vi "ConfigXMLCore.vi"(9 "ConnectionData":T1, 10 "controlsToSave":refnum<vi>[](array[refnum]), 11 "ConfigXMLControl":T2) -> ()   [LabVIEW 2015]
uses:
  ConfigXMLControl.ctl
  General/RemoteFiles/connectionData.ctl
panel:
  out "robotIP":string
  # "Core controller VI for the XML config plugin.\nhandles all saving, loading, file transfer, etc."
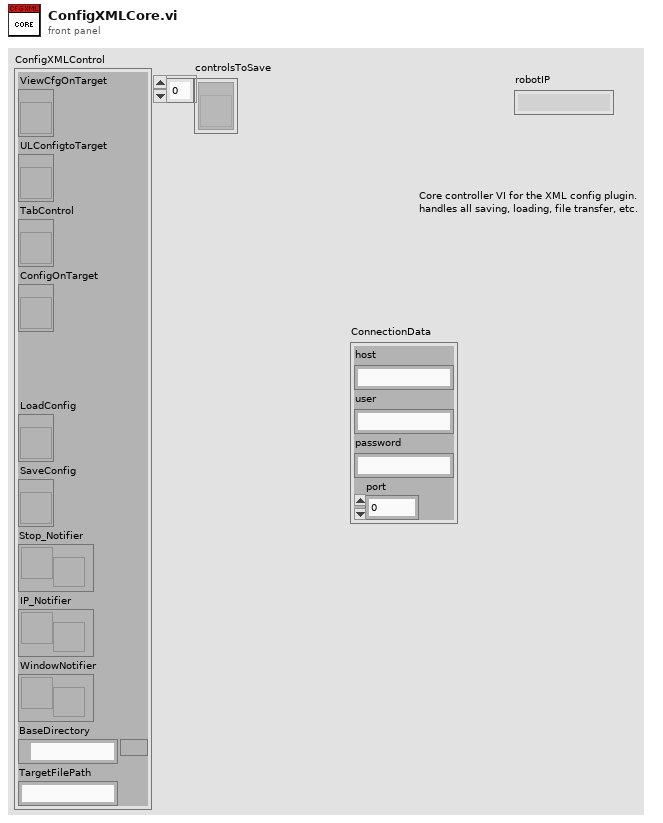
[diagram p1: front panel]
types:
  T1 = typedef "connectionData.ctl" = cluster{"host":string, "user":string, "password":string, "port":u16}
  T2 = typedef "ConfigXMLControl.ctl" = cluster{"ViewCfgOnTarget":refnum<vi>, "ULConfigtoTarget":refnum<vi>, "TabControl":refnum<vi>, "ConfigOnTarget":refnum<vi>, "LoadConfig":refnum<vi>, "SaveConfig":refnum<vi>, "Stop_Notifier":refnum<notifier>, "IP_Notifier":refnum<notifier>, "WindowNotifier":refnum<notifier>, "BaseDirectory":path, "TargetFilePath":string}
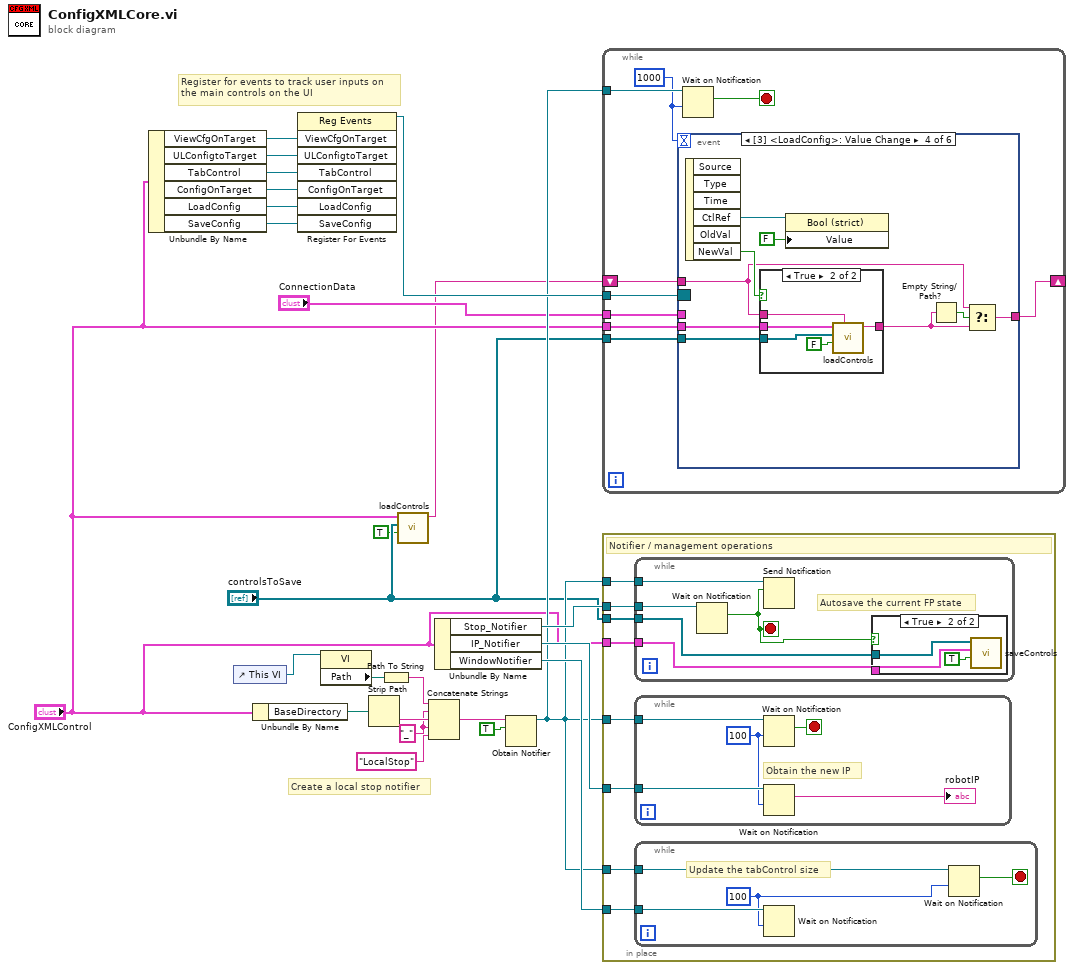
[diagram p0: block diagram]
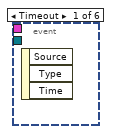
[diagram p3: hidden frame]
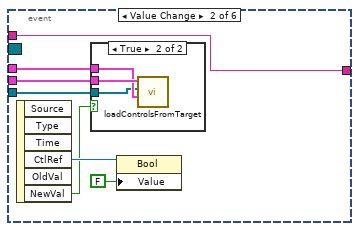
[diagram p4: hidden frame]
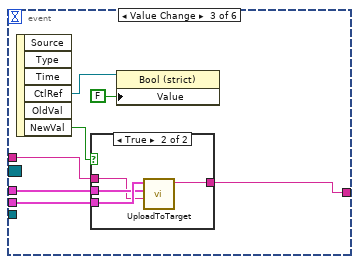
[diagram p6: hidden frame]
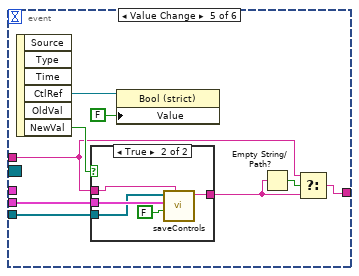
[diagram p9: hidden frame]
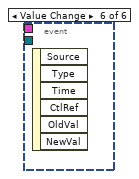
[diagram p11: hidden frame]
diagram:
  w10 = "_" ("string")
  # "Create a local stop notifier"
  # "Register for events to track user inputs on\nthe main controls on the UI"
  n1 = Unbundle By Name("ConfigXMLControl") -> ("ViewCfgOnTarget"=w22:refnum<vi>, "ULConfigtoTarget"=w21:refnum<vi>, "TabControl"=w20:refnum<vi>, "ConfigOnTarget"=w19:refnum<vi>, "LoadConfig"=w18:refnum<vi>, "SaveConfig"=w17:refnum<vi>)
  n2 = control-ref of="This VI"() -> (w15:refnum<vi>)
  n3 = Unbundle By Name("ConfigXMLControl") -> ("BaseDirectory"=w13:path)
  n4 = register-events(w22, w21, w20, w19, w18, w17) -> (reference out=w16:refnum<event-registration>)  [unwired: 2 in, 1 out]
  n5 = property class="VI"(reference=w15) -> ("Path"=w14:path)  [unwired: 1 in, 2 out]
  n6 = Strip Path(path=w13) -> (name=w11:string)  [unwired: 1 out]
  n7 = Path To String(path=w14) -> (string=w12:string)
  n8 = call "loadControls.vi"("Autoload?"=TRUE, "ControlsToLoad"="controlsToSave", "ConfigXMLControls"="ConfigXMLControl") -> ("nameUsed"=w2:string)  [unwired: 7 in, 1 out]
  n9 = Concatenate Strings(w12, w10, w11, w10, "LocalStop" ("string")) -> (w8:string)
  n10 = Unbundle By Name("ConfigXMLControl") -> ("Stop_Notifier"=w25:refnum<notifier>, "IP_Notifier"=w24:refnum<notifier>, "WindowNotifier"=w23:refnum<notifier>)
  n11 = Obtain Notifier(name (unnamed)=w8, notification data type=TRUE) -> (notifier out=w6:refnum<notifier>)  [unwired: 2 in, 2 out]
  n12 = while {
    tunnel: w16 -> [w34]
    tunnel: "ConfigXMLControl" -> [w33]
    tunnel: "controlsToSave" -> [w32]
    tunnel: w6 -> [w30]
    shift-right: [w28] -> _
    shift-left: w2 -> [w29]
    tunnel: "ConnectionData" -> [w27]
    stop <- w31 stop-if-true
    w26 = 1000
    n13 = event shown="[3] <LoadConfig>: Value Change" {
      selector: w34 -> [_ _ _ _ _ _]
      dyn-events: _ -> [_ _ _ _ _ _]
      timeout: w26 -> [_ _ _ _ _ _]
      tunnel: w33 -> [_ w38 w48 w63 w76 _]
      tunnel: w32 -> [_ w36 _ w64 w75 _]
      tunnel: w29 -> [_ w35 w46 w58 w71 _]
      tunnel: [_ w35 w45 w57 w72 _] -> w28
      tunnel: w27 -> [_ w37 w47 _ _ _]
      event Timeout {
        n14 = event-data() -> ()  [unwired: 1 in, 3 out]
      }
      event Value Change {
        n15 = event-data() -> ("CtlRef"=w40:refnum<vi>, "NewVal"=w39:bool)  [unwired: 1 in, 4 out]
        n16 = case shown="True" w39 {
          tunnel: w38 -> [_ w44]
          tunnel: w37 -> [_ w43]
          tunnel: w36 -> [_ w42]
          frame False {
          }
          frame True {
            n17 = call "loadControlsFromTarget.vi"("ConnectionData"=w43, "ControlsToLoad"=w42, "ConfigXMLControls"=w44) -> ()  [unwired: 8 in, 1 out]
          }
        }
        n18 = property class="Bool"(reference=w40, "Value"=FALSE) -> ()  [unwired: 1 in, 2 out]
      }
      event Value Change {
        n19 = event-data() -> ("CtlRef"=w51:refnum<vi>, "NewVal"=w49:bool)  [unwired: 1 in, 4 out]
        n20 = case shown="True" w49 {
          tunnel: w48 -> [_ w56]
          tunnel: w47 -> [_ w55]
          tunnel: w46 -> [w52 w54]
          tunnel: [w52 w53] -> w45
          frame False {
          }
          frame True {
            n21 = call "UploadToTarget.vi"("previousName"=w54, "ConnectionData"=w55, "ConfigXMLControls"=w56) -> ("newName"=w53:string)  [unwired: 7 in, 1 out]
          }
        }
        n22 = property class="Bool (strict)"(reference=w51, "Value"=FALSE) -> ()  [unwired: 1 in, 2 out]
      }
      event Value Change {
        n23 = event-data() -> ("CtlRef"=w62:refnum<vi>, "NewVal"=w61:bool)  [unwired: 1 in, 4 out]
        n24 = case shown="True" w61 {
          tunnel: w63 -> [_ w68]
          tunnel: w64 -> [_ w70]
          tunnel: [_ w67] -> w59
          tunnel: w58 -> [_ w66]
          frame False {
          }
          frame True {
            n25 = call "loadControls.vi"("prevName"=w66, "Autoload?"=FALSE ("isAutoSave"), "ControlsToLoad"=w70, "ConfigXMLControls"=w68) -> ("nameUsed"=w67:string)  [unwired: 6 in, 1 out]
          }
        }
        n26 = property class="Bool (strict)"(reference=w62, "Value"=FALSE) -> ()  [unwired: 1 in, 2 out]
        n27 = Empty String/Path?(string/path=w59) -> (empty?=w60:bool)
        n28 = Select(t=w58, s=w60, f=w59) -> (s? t:f=w57:string)
      }
      event Value Change {
        n29 = event-data() -> ("CtlRef"=w79:refnum<vi>, "NewVal"=w77:bool)  [unwired: 1 in, 4 out]
        n30 = case shown="True" w77 {
          tunnel: w76 -> [_ w84]
          tunnel: w75 -> [_ w83]
          tunnel: [_ w81] -> w73
          tunnel: w71 -> [_ w80]
          frame False {
          }
          frame True {
            n31 = call "saveControls.vi"("prevName"=w80, "isAutoSave"=FALSE, "ConfigXMLControls"=w84, "ControlsToSave"=w83) -> ("nameUsed"=w81:string)  [unwired: 6 in, 1 out]
          }
        }
        n32 = property class="Bool (strict)"(reference=w79, "Value"=FALSE) -> ()  [unwired: 1 in, 2 out]
        n33 = Empty String/Path?(string/path=w73) -> (empty?=w74:bool)
        n34 = Select(t=w71, s=w74, f=w73) -> (s? t:f=w72:string)
      }
      event Value Change {
        n35 = event-data() -> ()  [unwired: 1 in, 6 out]
      }
    }
    n36 = Wait on Notification(notifier=w30, timeout in ms (-1)=w26) -> (notification=w31:bool)  [unwired: 2 in, 3 out]
  }
  n37 = in-place {
    in-place-border: w25 -> [w92]
    in-place-border: w24 -> [w91]
    in-place-border: w23 -> [w90]
    in-place-border: "ConfigXMLControl" -> [w89]
    in-place-border: "controlsToSave" -> [w88]
    in-place-border: w6 -> [w87]
    in-place-border: w6 -> [w86]
    in-place-border: w6 -> [w85]
    # "Notifier / management operations"
    n38 = while {
      tunnel: w92 -> [w106]
      tunnel: w89 -> [w105]
      tunnel: w88 -> [w104]
      tunnel: w87 -> [w103]
      stop <- w102 stop-if-true
      # "Autosave the current FP state"
      n39 = Wait on Notification(notifier=w106) -> (notification=w102:bool)  [unwired: 3 in, 3 out]
      n40 = Send Notification(notification=w102, notifier=w103) -> ()  [unwired: 1 in, 2 out]
      n41 = case shown="True" w102 {
        tunnel: w105 -> [_ w109]
        tunnel: w104 -> [_ w108]
        frame False {
        }
        frame True {
          n42 = call "saveControls.vi"("isAutoSave"=TRUE, "ConfigXMLControls"=w109, "ControlsToSave"=w108) -> ()  [unwired: 7 in, 2 out]
        }
      }
    }
    n43 = while {
      tunnel: w91 -> [w101]
      tunnel: w86 -> [w99]
      stop <- w98 stop-if-true
      w97 = 100 ("timeout in ms (-1)")
      # "Obtain the new IP"
      n44 = Wait on Notification(notifier=w99, timeout in ms (-1)=w97) -> (notification=w98:bool)  [unwired: 2 in, 3 out]
      n45 = Wait on Notification(notifier=w101, timeout in ms (-1)=w97) -> (notification=→"robotIP":string)  [unwired: 2 in, 3 out]
    }
    n46 = while {
      tunnel: w90 -> [w96]
      tunnel: w85 -> [w94]
      stop <- w93 stop-if-true
      w95 = 100 ("timeout in ms (-1)")
      # "Update the tabControl size"
      n47 = Wait on Notification(notifier=w96, timeout in ms (-1)=w95) -> ()  [unwired: 2 in, 4 out]
      n48 = Wait on Notification(notifier=w94, timeout in ms (-1)=w95) -> (notification=w93:bool)  [unwired: 2 in, 3 out]
    }
  }
